vi "Launch Plugin (Info).vi"(8 "error in (no error)":errorcluster, 10 "Plugin Info":T1, 11 "GUI Manager Module in":refnum<class "GUI Manager Module.lvclass">) -> (0 "error out":errorcluster, 3 "GUI Manager Module out":refnum<class "GUI Manager Module.lvclass">)   [LabVIEW 2020, in "VolatusGUI.lvlib" / "GUI Manager Module.lvclass"]
uses:
  GUI Manager Module.lvclass
  C:/dev/lv20CE/relink/lv-volatus/Volatus/Module/Module.lvclass
  Plugin Info.ctl
  VolatusConfig/Meta Name.ctl
  PluginGUI/PluginGUI.lvclass
  Volatus/Module/Module.lvclass
  Volatus/Module/Module.lvclass/Module.ctl
  Volatus/VolatusAPI/VolatusAPI.lvclass/VolatusAPI.ctl
  VolatusConfig/VolatusConfigElement/VolatusConfigElement.lvclass/VolatusConfigElement.ctl
  VolatusConfig/VolatusConfigElement/Element.vi
  VolatusConfig/Node/Node.lvclass
  C:/dev/lv20CE/relink/lv-volatus/VolatusConfig/VolatusConfigElement/VolatusConfigElement.lvclass
  VolatusConfig/Task/Task.lvclass
  lv-cdm/CDM-Config/Config Lookup/Match Meta.vi
  lv-cdm/CDM-Config/Config Element/Owner.vi
  lv-cdm/CDM-Config/Config Manager/Lookup Descendant.vi
  lv-cdm/CDM-Config/Config Filter/Config Lookup.lvclass
  GUI Manager Module.lvclass/GUI Manager Module.ctl
  VolatusConfig/VolatusConfig.lvlib
  Volatus/VolatusAPI/VolatusAPI.lvclass
  VolatusConfig/VolatusConfigElement/VolatusConfigElement.lvclass
  C:/dev/lv20CE/relink/lv-volatus/VolatusGUI/GUI Manager Module/GUI Manager Module.lvclass
  C:/dev/lv20CE/relink/lv-volatus/VolatusGUI/PluginGUI/PluginGUI.lvclass
  Volatus/Volatus.lvlib
  C:/dev/lv20CE/relink/lv-volatus/VolatusConfig/Task/Task.lvclass
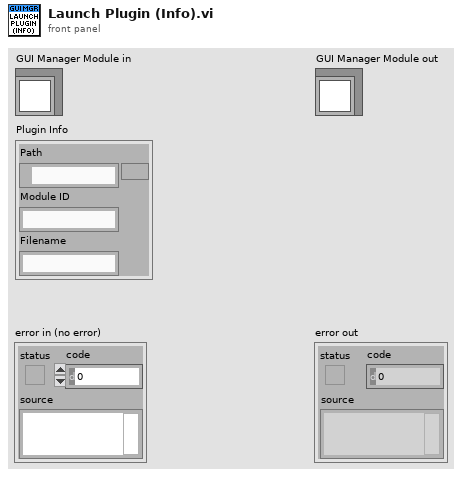
[diagram p1: front panel]
types:
  T1 = typedef "VolatusGUI.lvlib/GUI Manager Module.lvclass/Plugin Info.ctl" = cluster{"Path":path, "Module ID":string, "Filename":string}
  T2 = typedef "VolatusConfig.lvlib/Meta Name.ctl" = enum16{"VL_Type", "VL_Node_IP", "VL_Node_Type", "VL_Task_Type", "VL_Group_Type", "VL_Channel_Type", "VL_Channel_DataType", "VL_Config_Version", "VL_Overlay_Type", "VL_Config_Hash"}
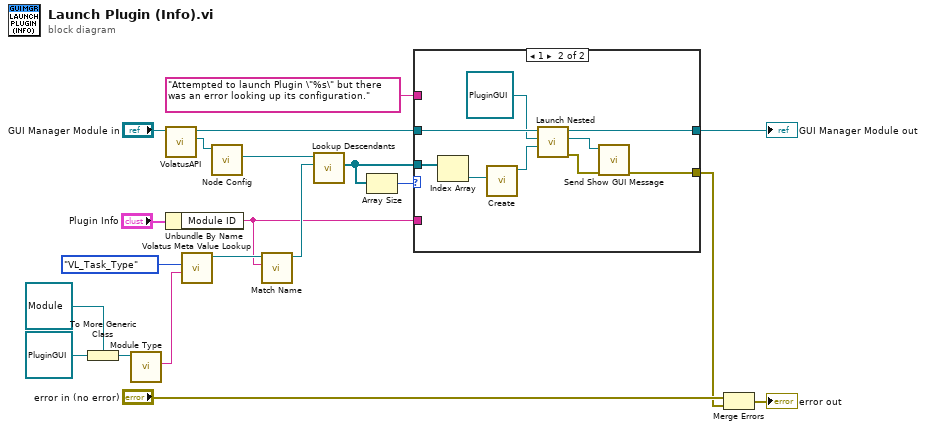
[diagram p0: block diagram]
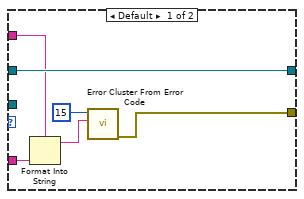
[diagram p2: hidden frame]
diagram:
  n1 = To More Generic Class(target class=refnum<class "Module.lvclass"> refnum ("Volatus:Module"), reference=refnum<class "PluginGUI.lvclass"> refnum ("VolatusGUI:PluginGUI.lvclass")) -> (generic class reference=w14:refnum<class "Module.lvclass">)
  n2 = call-dynamic "Module Type.vi"("Module in"=w14) -> ("Module Type"=w12:string)  [unwired: 10 in]
  n3 = call "VolatusAPI.vi"("Module in"="GUI Manager Module in") -> ("VolatusAPI"=w18:refnum<class "VolatusAPI.lvclass">, "Module out"=w6:refnum<class "GUI Manager Module.lvclass">)  [unwired: 9 in]
  n4 = Unbundle By Name("Plugin Info") -> ("Module ID"=w4:string)
  n5 = call "Volatus Meta Value Lookup.vi"("Value"=w12, "Meta Name"=Meta_Name."VL_Task_Type") -> ("Config Lookup out"=w11:refnum<class "Config Lookup.lvclass">)  [unwired: 8 in, 1 out]
  n6 = call "Node Config.vi"("VolatusAPI in"=w18) -> ("Node Config"=w16:refnum<class "Node.lvclass">)  [unwired: 9 in, 1 out]
  n7 = call "Match Name.vi"("Name"=w4, "Config Lookup (New)"=w11) -> ("Config Lookup out"=w9:refnum<class "Config Lookup.lvclass">)  [unwired: 8 in, 1 out]
  n8 = call "Lookup Descendants.vi"("Lookup"=w9, "VolatusConfigElement in"=w16) -> ("Descendants"=w8:refnum<class "Config Element.lvclass">[])  [unwired: 7 in, 2 out]
  n9 = Array Size(array=w8) -> (size(s)=w7:i32)
  n10 = case shown="1" w7 {
    tunnel: w8 -> [_ w35]
    tunnel: w6 -> [w26 w33]
    tunnel: [w26 w32] -> w5
    tunnel: [w25 w27] -> w1
    tunnel: w4 -> [w22 _]
    tunnel: "Attempted to launch Plugin \"%s\" but there was an error looking up its configuration." -> [w23 _]
    frame Default {
      n11 = Format Into String(format string=w23, w22) -> (resulting string=w21:string)  [unwired: 2 in, 1 out]
      n12 = call <vilib>:"Error Cluster From Error Code.vi"("error message (\"\")"=w21, "error code (0)"=15) -> ("error out"=w25:errorcluster)  [unwired: 7 in]
    }
    frame 1 {
      n13 = Index Array(array=w35) -> (element=w34:refnum<class "Config Element.lvclass">)  [unwired: 1 in]
      n14 = call "Create.vi"("Element"=w34) -> ("Task out"=w31:refnum<class "Task.lvclass">)  [unwired: 9 in, 1 out]
      n15 = call "Launch Nested.vi"("Config Element"=w31, "Nested Module"=refnum<class "PluginGUI.lvclass"> refnum ("VolatusGUI:PluginGUI.lvclass"), "Parent in"=w33) -> ("error out"=w29:errorcluster, "MessageQ"=w28:refnum<class "MessageQ.lvclass">, "Parent out"=w32:refnum<class "GUI Manager Module.lvclass">)  [unwired: 6 in]
      n16 = call "Send Show GUI Message.vi"("error in (no error)"=w29, "MessageQ"=w28) -> ("error out"=w27:errorcluster)  [unwired: 9 in]
    }
  }
  "GUI Manager Module out" <- w5
  n17 = Merge Errors("error in (no error)", w1) -> (→"error out":errorcluster)
